vi "20170321-lecture3-2 c.vi"() -> ()   [LabVIEW 2014]
panel:
  out "Numeric":i32
  out "number: 0 to 1":dbl
  in  "stop":bool
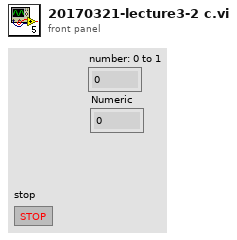
[diagram p1: front panel]
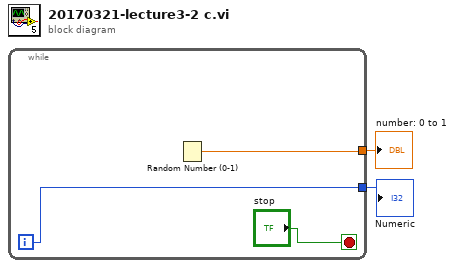
[diagram p0: block diagram]
diagram:
  n1 = while {
    tunnel: [w4] -> w2
    tunnel: [w3] -> w1
    i -> [w3]
    stop <- "stop" stop-if-true
    n2 = Random Number (0-1)() -> (number: 0 to 1=w4:dbl)
  }
  "number: 0 to 1" <- w2
  "Numeric" <- w1
